vi "midiOutPlayer.msg.Resume.vi"(8 "error in (no error)":errorcluster, 11 "midiPlayer in":refnum<class "midiPlayer.lvclass">) -> (0 "error out":errorcluster, 3 "midiPlayer out":refnum<class "midiPlayer.lvclass">)   [LabVIEW 2020, in "midiPlayer.lvclass"]
uses:
  midiPlayer.lvclass
  midiPlayer.lvclass/midiPlayer.ctl
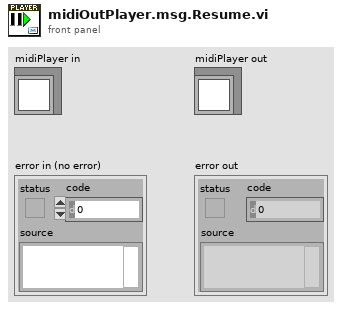
[diagram p1: front panel]
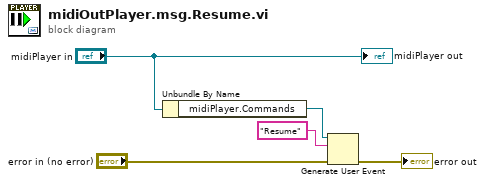
[diagram p0: block diagram]
diagram:
  n1 = Unbundle By Name("midiPlayer in") -> ("midiPlayer.Commands"=w5:refnum<user-event>)
  n2 = Generate User Event(user event=w5, event data cluster="Resume" ("event data"), error in="error in (no error)") -> (error out=→"error out":errorcluster)  [unwired: 1 in, 1 out]
  "midiPlayer out" <- "midiPlayer in"
